vi "test Detects Missing Required Options.vi"(8 "error in (no error)":errorcluster, 11 "TestCase in":refnum<class "Options Parsing Tests.lvclass">) -> (0 "error out":errorcluster, 3 "TestCase out":refnum<class "Options Parsing Tests.lvclass">)   [LabVIEW 2011, in "Options Parsing Tests.lvclass"]
uses:
  Options Parsing Tests.lvclass
  Argument Parser/Option Class/Option Configuration.ctl
  Argument Parser/Option Class/Argument Type.ctl
  <vilib>/addons/_JKI Toolkits/VI Tester/TestCase.llb/TestCase.lvclass
  Argument Parser/Option Set Class/Option Set.lvclass
  Argument Parser/Option Class/Option.lvclass
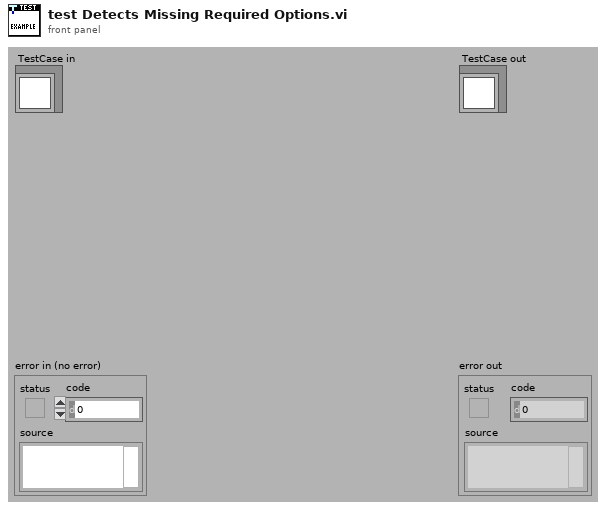
[diagram p1: front panel]
types:
  T1 = typedef "Option Parser.lvlib/Option.lvclass/Option Configuration.ctl" = cluster{"Option Type":T2, "Option Labels":string[], "Key":string, "Description":string, "Required":bool, "Default Value":string}
  T2 = typedef "Option Parser.lvlib/Option.lvclass/Argument Type.ctl" = enum16{"flag", "value"}
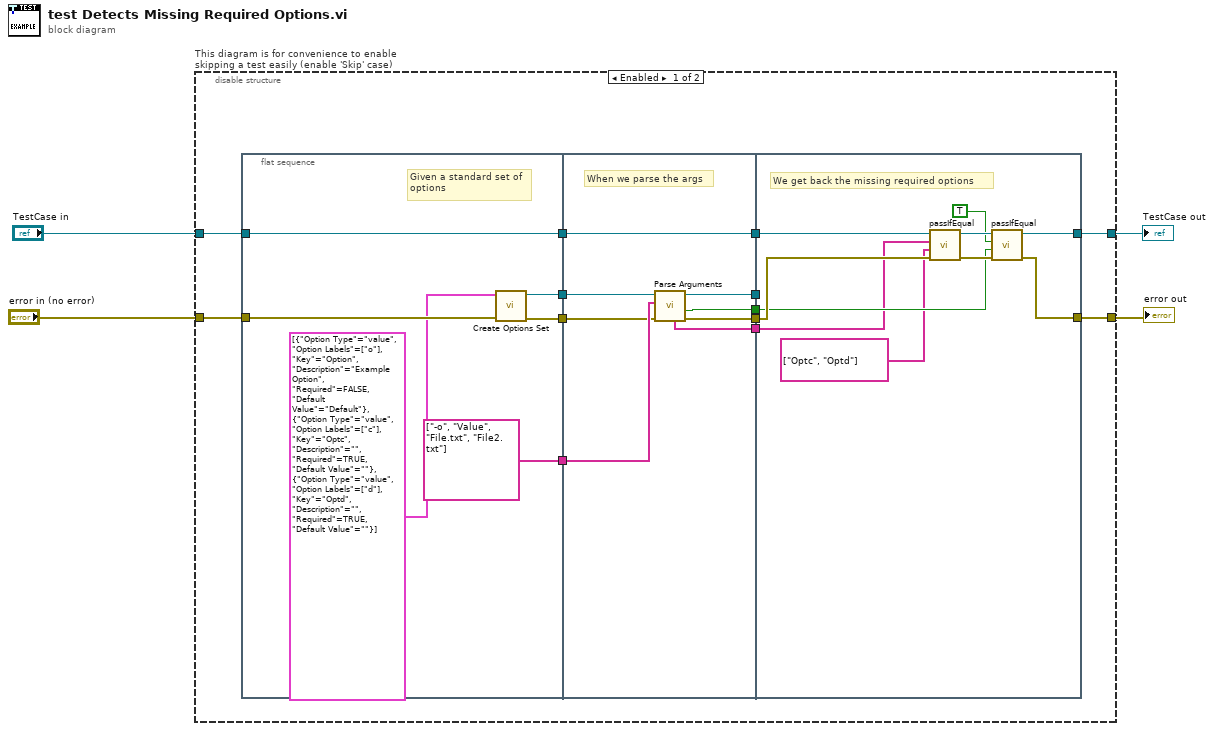
[diagram p0: block diagram]
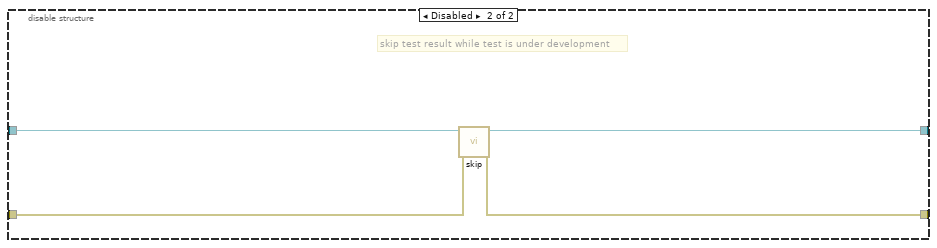
[diagram p2: hidden frame]
diagram:
  n1 = disable-structure "This diagram is for convenience to enable skipping a test easily (enable 'Skip' case)" shown="Enabled" {
    disable-tunnel: "TestCase in" -> [w9 w45]
    disable-tunnel: [w8 w43] -> w1
    disable-tunnel: [w7 w44] -> w3
    disable-tunnel: "error in (no error)" -> [w16 w42]
    frame Enabled {
      n2 = flat-sequence {
        tunnel: [string[] ["-o", "Value", "File.txt", "File2.txt"]] -> w17
        tunnel: w16 -> [w22]
        tunnel: [w21] -> w15
        tunnel: [w20] -> w14
        tunnel: [w19] -> w10
        tunnel: w9 -> [w19]
        tunnel: w17 -> [w31]
        tunnel: w15 -> [w30]
        tunnel: w14 -> [w29]
        tunnel: [w28] -> w13
        tunnel: [w27] -> w12
        tunnel: [w26] -> w11
        tunnel: w10 -> [w26]
        tunnel: [w25] -> w6
        tunnel: [w24] -> w5
        tunnel: w13 -> [_]
        tunnel: w12 -> [w41]
        tunnel: w11 -> [w40]
        tunnel: [w36] -> w8
        tunnel: [w38] -> w7
        tunnel: w6 -> [w35]
        tunnel: w5 -> [w34]
        frame #0 {
          # "Given a standard set of\noptions"
          n3 = call "Create Options Set.vi"("error in (no error)"=w22, "Options"=T1[] [{"Option Type"=enum."value", "Option Labels"=["o"], "Key"="Option", "Description"="Example Option", "Required"=FALSE, "Default Value"="Default"}, {"Option Type"=enum."value", "Option Labels"=["c"], "Key"="Optc", "Description"="", "Required"=TRUE, "Default Value"=""}, {"Option Type"=enum."value", "Option Labels"=["d"], "Key"="Optd", "Description"="", "Required"=TRUE, "Default Value"=""}]) -> ("error out"=w21:errorcluster, "Option Set out"=w20:refnum<class "Option Set.lvclass">)  [unwired: 8 in]
        }
        frame #1 {
          # "When we parse the args"
          n4 = call "Parse Arguments.vi"("error in (no error)"=w30, "Arguments"=w31, "Option Set in"=w29) -> ("error out"=w27:errorcluster, "Missing Options"=w25:bool, "Option Set out"=w28:refnum<class "Option Set.lvclass">, "Missing Option Keys"=w24:string[])  [unwired: 5 in]
        }
        frame #2 {
          # "We get back the missing required options"
          n5 = call-dynamic "passIfEqual.vi"("error in (no error)"=w41, "y"=string[] ["Optc", "Optd"] ("Missing Option Keys"), "x"=w34, "TestCase in"=w40) -> ("error out"=w39:errorcluster, "TestCase out"=w37:refnum<class "Options Parsing Tests.lvclass">)  [unwired: 6 in]
          n6 = call-dynamic "passIfEqual.vi"("error in (no error)"=w39, "y"=w35, "x"=TRUE ("Missing Options"), "TestCase in"=w37) -> ("error out"=w38:errorcluster, "TestCase out"=w36:refnum<class "Options Parsing Tests.lvclass">)  [unwired: 6 in]
        }
      }
    }
    frame Disabled {
      # "skip test result while test is under development"
      n7 = call <vilib>:"skip.vi"("error in (no error)"=w42, "TestCase in"=w45) -> ("error out"=w44:errorcluster, "TestCase out"=w43:refnum<class "Options Parsing Tests.lvclass">)  [unwired: 8 in]
    }
  }
  "error out" <- w3
  "TestCase out" <- w1
